vi "S2DS- External Write-Check.vi"() -> ()   [LabVIEW 2016]
doc: "Uses DataSocket to read array data. \n \nThe Writer, Server, and Reader can all be on the same computer or different computers. The Writer and Reader URLs should point to the computer where the DataSocket Server is."
panel:
  in  "Number identifier":i32
  out "data":dbl
  in  "Stop":bool
  # "Overview: Demonstrates the use of the DataSocket functions to read data from the DataSocket server of S2DS.\nRequirements: Windows\nInstructions:\n1. Ensure Simple 2D Sweep : Export data  is TRUE.\n2. Run the VI.\n3. Click Stop to stop the VI."
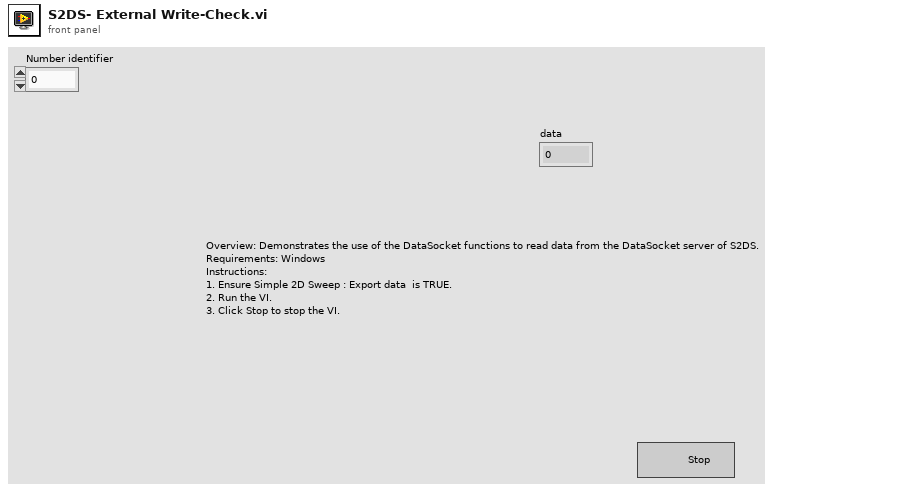
[diagram p1: front panel]
types:
  T1 = enum16{"Read", "Write", "ReadWrite", "BufferedRead", "BufferedReadWrite"}
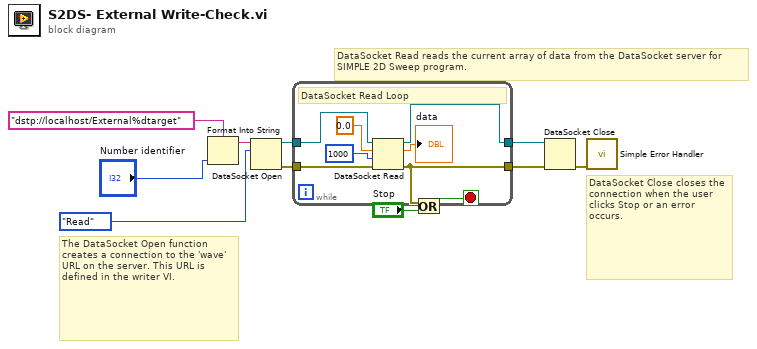
[diagram p0: block diagram]
diagram:
  # "The DataSocket Open function creates a connection to the 'wave' URL on the server. This URL is defined in the writer VI."
  # "DataSocket Read reads the current array of data from the DataSocket server for SIMPLE 2D Sweep program."
  # "DataSocket Close closes the connection when the user clicks Stop or an error occurs."
  n1 = Format Into String(format string="dstp://localhost/External%dtarget" ("Write Location"), "Number identifier") -> (resulting string=w1:string)  [unwired: 2 in, 1 out]
  n2 = DataSocket Open(10:T1."Read" ("mode"), 11:w1) -> (0:w9:errorcluster, 3:w4:refnum<k13>)  [unwired: 2 in]
  n3 = while {
    tunnel: [w13] -> w8
    tunnel: w9 -> [w15]
    tunnel: w4 -> [w16]
    tunnel: [w12] -> w5
    stop <- w17 stop-if-true
    # "DataSocket Read Loop"
    n4 = DataSocket Read(8:w15, 9:1000 ("ms timeout (10000)"), 10:0.0, 11:w16) -> (0:w13:errorcluster, 2:→"data":dbl, 3:w12:refnum<k13>)  [unwired: 5 out]
    n5 = Or(x=w13, y="Stop") -> (x .or. y?=w17:bool)
  }
  n6 = DataSocket Close(8:w8, 11:w5) -> (0:w6:errorcluster)  [unwired: 1 in, 1 out]
  n7 = call <vilib>:"Simple Error Handler.vi"("error in (no error)"=w6) -> ()  [unwired: 4 in, 5 out]
